vi "LTVDiffDriveCtrl_Calculate_TrajState.vi"(6 "DesiredState":T1={"TimeSeconds"=0.0, "Velocity"=0.0, "Acceleration"=0.0, "POSE"={"TRANSLATION"={"X"=0.0, "Y"=0.0}, "ROTATION"={"VALUE"=0.0, "COS"=1.0, "SIN"=0.0}}, "Curvature"=0.0} {"POSE"."ROTATION"."SIN" format="%13.4f"; "POSE"."ROTATION"."COS" format="%13.4f"; "POSE"."ROTATION"."VALUE" format="%13.4f"; "POSE"."TRANSLATION"."Y" format="%14.3f"; "POSE"."TRANSLATION"."X" format="%14.3f"}, 8 "Right Velocity":dbl, 9 "Left Velocity":dbl, 10 "CurrentPose":T2={"TRANSLATION"={"X"=0.0, "Y"=0.0}, "ROTATION"={"VALUE"=0.0, "COS"=1.0, "SIN"=0.0}} {"ROTATION"."SIN" format="%13.4f"; "ROTATION"."COS" format="%13.4f"; "ROTATION"."VALUE" format="%13.4f"; "TRANSLATION"."Y" format="%14.3f"; "TRANSLATION"."X" format="%14.3f"}, 11 "in LTVDiffDrveCtrl":T5) -> (0 "Error":bool, 1 "Right Voltage":dbl, 2 "Left Voltage":dbl, 3 "out LTVDiffDriveCtrl":T5)   [LabVIEW 2019, in "Trajectory_Library.lvlib"]
doc: "Create implicit model follower\n\nInputs:\n - A < states, states > -- Continuous system matrix of the plant being controlled.\n - B < states, inputs > -- Continuous input matrix of the plant being controlled.\n - A_Ref < states, states > -- Continuous system matrix whose dymanics should be followed.\n - B_Ref < states, inputs > -- Continuous input matrix x whose dymanics should be followed.\n\nOutputs:\n - Error -- If TRUE, an error occured."
uses:
  Trajectory_Library.lvlib
  TypeDef/LTV_DIFF_DRIVE_CTRL.ctl
  TypeDef/FUNCTION_GENERATOR_MATRIX.ctl
  <vilib>/Analysis/Matrix/Datatypes/RealMatrix.ctl
  POSE2D.ctl
  TRANSLATION2D.ctl
  ROTATION2D.ctl
  TRAJ_STATE.ctl
  <vilib>/Analysis/Matrix/NI_Matrix.lvlib
panel:
  # "< 5, 1 >"
  # "< 5, 1 >"
  # "< 5, 1 >"
  # "< 5, 1 >"
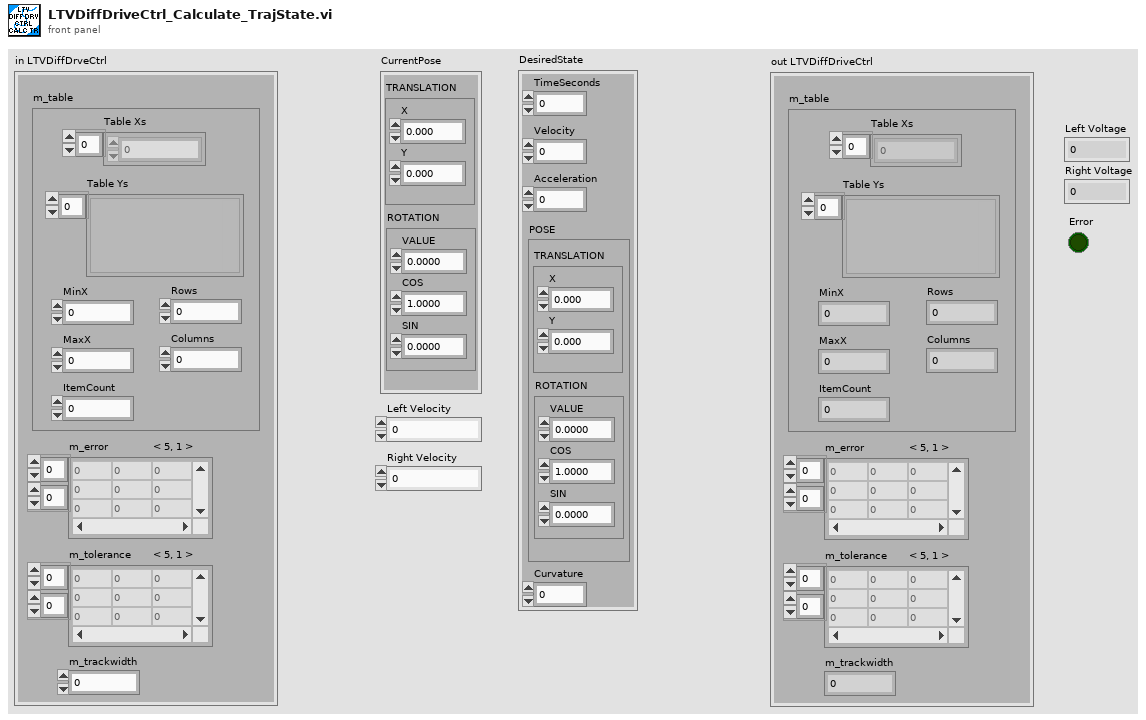
[diagram p1: front panel]
types:
  T1 = typedef "Trajectory_Library.lvlib/TRAJ_STATE.ctl" = cluster{"TimeSeconds":dbl, "Velocity":dbl, "Acceleration":dbl, "POSE":T2, "Curvature":dbl}
  T2 = typedef "Trajectory_Library.lvlib/POSE2D.ctl" = cluster{"TRANSLATION":T3, "ROTATION":T4}
  T3 = typedef "Trajectory_Library.lvlib/TRANSLATION2D.ctl" = cluster{"X":dbl, "Y":dbl}
  T4 = typedef "Trajectory_Library.lvlib/ROTATION2D.ctl" = cluster{"VALUE":dbl, "COS":dbl, "SIN":dbl}
  T5 = typedef "Trajectory_Library.lvlib/LTV_DIFF_DRIVE_CTRL.ctl" = cluster{"m_table":T6, "m_error":T7, "m_tolerance":T7, "m_trackwidth":dbl}
  T6 = typedef "Trajectory_Library.lvlib/FUNCTION_GENERATOR_MATRIX.ctl" = cluster{"Table Xs":dbl[], "Table Ys":variant[], "MinX":dbl, "MaxX":dbl, "ItemCount":i32, "Rows":i32, "Columns":i32}
  T7 = typedef "NI_Matrix.lvlib/RealMatrix.ctl" = dbl[][]
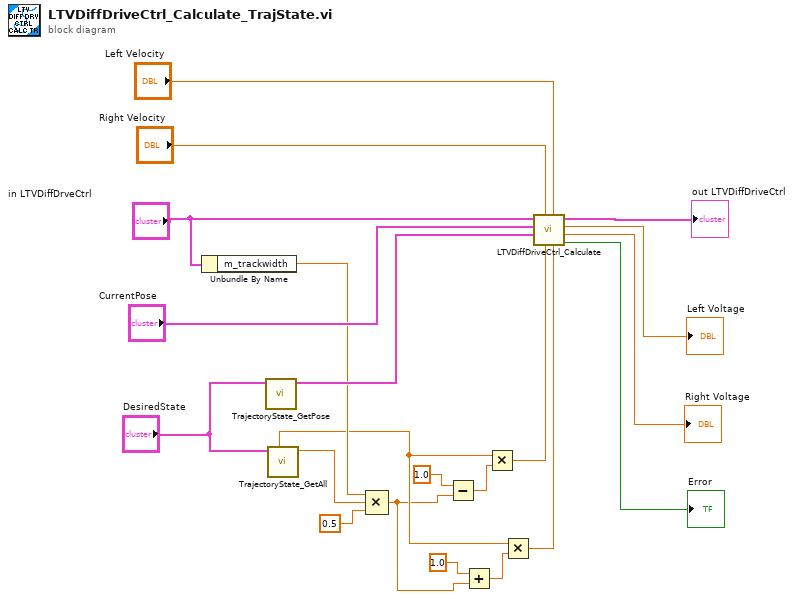
[diagram p0: block diagram]
diagram:
  n1 = Unbundle By Name("in LTVDiffDrveCtrl") -> ("m_trackwidth"=w12:dbl)
  n2 = call "TrajectoryState_GetPose.vi"("TRAJ_STATE"="DesiredState") -> ("TrajStatePose"=w17:T2)  [unwired: 10 in]
  n3 = call "TrajectoryState_GetAll.vi"("TRAJ_STATE"="DesiredState") -> ("Curvature"=w11:dbl, "Velocity"=w7:dbl)  [unwired: 4 in, 5 out]
  n4 = Compound Arithmetic op=MULTIPLY(w12, w11, 0.5 ("value")) -> (w6:dbl)
  n5 = Subtract(x=1.0, y=w6) -> (x-y=w10:dbl)
  n6 = Add(x=1.0, y=w6) -> (x+y=w8:dbl)
  n7 = Multiply(x=w7, y=w10) -> (x*y=w5:dbl)
  n8 = Multiply(x=w7, y=w8) -> (x*y=w4:dbl)
  n9 = call "LTVDiffDriveCtrl_Calculate.vi"("Ref Right Velocity"=w4, "Left Velocity"="Left Velocity", "Ref Left Velocity"=w5, "Right Velocity"="Right Velocity", "RefPose"=w17, "CurrentPose"="CurrentPose", "in LTVDiffDriveCtrl"="in LTVDiffDrveCtrl") -> ("Error"=→"Error":bool, "Right Voltage"=→"Right Voltage":dbl, "Left Voltage"=→"Left Voltage":dbl, "out LTVDiffDriveCtrl"=→"out LTVDiffDriveCtrl":T5)  [unwired: 1 in]
